vi "Delete Database.vi"(0 "InfluxDB in":refnum<class "InfluxDB Client.lvclass">, 5 "Database name":string, 11 "error in (no error)":errorcluster) -> (4 "InfluxDB out":refnum<class "InfluxDB Client.lvclass">, 15 "error out":errorcluster)   [LabVIEW 2017]
doc: "Deletes a database."
uses:
  <vilib>/httpClient/LabVIEWHTTPClient.lvlib
  InfluxDB Client.lvclass
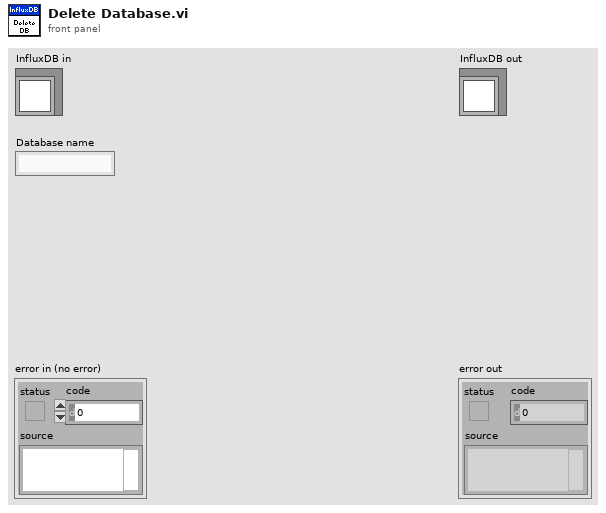
[diagram p1: front panel]
types:
  T1 = typedef "LabVIEWHTTPClient.lvlib/ClientHandle.ctl" = refnum<k1>
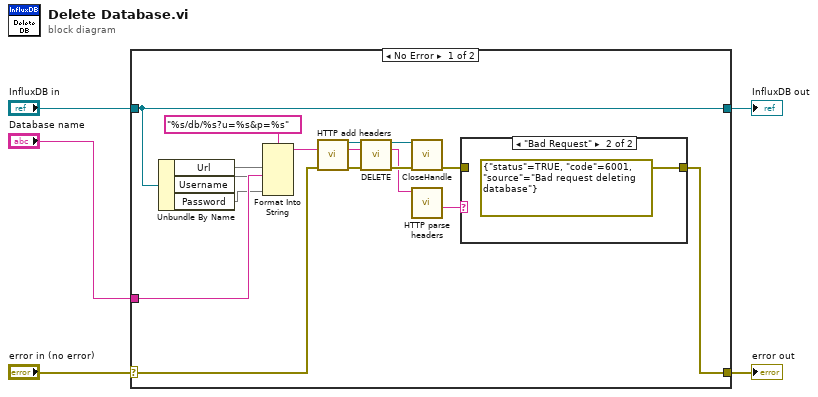
[diagram p0: block diagram]
diagram:
  n1 = case shown="No Error" "error in (no error)" {
    selector: "error in (no error)" -> [w8 w25]
    tunnel: [w9 w25] -> w4
    tunnel: [w21 w24] -> w2
    tunnel: "InfluxDB in" -> [w21 w24]
    tunnel: "Database name" -> [w14 _]
    frame No Error {
      n2 = Unbundle By Name(w21) -> ("Url"=w19, "Username"=w13, "Password"=w12)
      n3 = Format Into String(format string="%s/db/%s?u=%s&p=%s" ("url"), w19, w14, w13, w12) -> (resulting string=w16:string)  [unwired: 2 in, 1 out]
      n4 = call "HTTP add headers.vi"("error in (no error)"=w8) -> ("client handle out"=w6:T1, "error out"=w7:errorcluster)  [unwired: 13 in]
      n5 = call <vilib>:"DELETE.vi"("client handle"=w6, "url"=w16, "error in (no error)"=w7) -> ("client handle out"=w18:T1, "headers"=w15:string, "error out"=w17:errorcluster)  [unwired: 9 in, 1 out]
      n6 = call <vilib>:"CloseHandle.vi"("client handle"=w18, "error in (no error)"=w17) -> ("error out"=w11:errorcluster)  [unwired: 13 in]
      n7 = call "HTTP parse headers.vi"("HTTP headers"=w15) -> ("Status"=w10:string)  [unwired: 8 in, 2 out]
      n8 = case shown="\"Bad Request\"" w10 {
        tunnel: w11 -> [w22 _]
        tunnel: [w22 errorcluster {"status"=TRUE, "code"=6001, "source"="Bad request deleting database"} ("error constant")] -> w9
        frame Default {
        }
        frame "Bad Request" {
        }
      }
    }
    frame Error {
    }
  }
  "error out" <- w4
  "InfluxDB out" <- w2
